vi "BoxExecute_ForSim.vi"(11 "Inputs":T5) -> (1 "OtherOutputs":T3={"ShootLOnTarg"=FALSE, "ShootROnTarg"=FALSE, "StateMachineState"=enum."initilization", "Box Note State"=enum."note in shooter wheels", "ShootR SP"=0.0, "ShootR FF"=0.0, "ShootR Filt RPM"=0.0, "ShootL SP"=0.0, "ShootL FF"=0.0, "ShootL Filt RPM"=0.0}, 3 "Outputs":T4)   [LabVIEW 2023]
uses:
  BoxStatesEnum.ctl
  BoxNoteState.ctl
  <vilib>/Rock Robotics/WPI/ThirdParty/JAS_Junk/TrajLib/TypeDef/PID_ERROR_TOLERANCE.ctl
  <vilib>/Rock Robotics/WPI/ThirdParty/JAS_Junk/TrajLib/LinearFilter_ResetToValue.vi
  <vilib>/Rock Robotics/WPI/ThirdParty/JAS_Junk/TrajLib/LinearFilter_Calculate.vi
  <vilib>/Rock Robotics/WPI/ThirdParty/JAS_Junk/TrajLib/VI/BoolCmd_Recv_Internal.vi
  <vilib>/Rock Robotics/WPI/ThirdParty/JAS_Junk/TrajLib/VI/DigSeqLogic_Edge_On.vi
  <vilib>/Rock Robotics/WPI/ThirdParty/JAS_Junk/TrajLib/SimpleMotorFF_Calculate.vi
  <vilib>/Rock Robotics/WPI/ThirdParty/JAS_Junk/TrajLib/PIDController_AtSetpoint.vi
  <vilib>/Rock Robotics/WPI/ThirdParty/JAS_Junk/TrajLib/PIDController_SetPIDF.vi
  <vilib>/Rock Robotics/WPI/ThirdParty/JAS_Junk/TrajLib/PIDController_SetDerivativeFilter.vi
  <vilib>/Rock Robotics/WPI/ThirdParty/JAS_Junk/TrajLib/PIDController_SetIntegratorRange.vi
  <vilib>/Rock Robotics/WPI/ThirdParty/JAS_Junk/TrajLib/PIDController_SetTolerancePandV.vi
  <vilib>/Rock Robotics/WPI/ThirdParty/JAS_Junk/TrajLib/PIDController_DisableContinousInput.vi
  <vilib>/Rock Robotics/WPI/ThirdParty/JAS_Junk/TrajLib/PIDController_EnableContinousInput.vi
  <vilib>/Rock Robotics/WPI/ThirdParty/JAS_Junk/TrajLib/PIDController_Reset.vi
  <vilib>/Rock Robotics/WPI/ThirdParty/JAS_Junk/TrajLib/PIDController_New.vi
  <vilib>/Rock Robotics/WPI/ThirdParty/JAS_Junk/TrajLib/PIDController_SetOutputLimits.vi
  <vilib>/Rock Robotics/WPI/ThirdParty/JAS_Junk/TrajLib/VI/BoolCmd_ObtainQueue.vi
  <vilib>/Rock Robotics/WPI/ThirdParty/JAS_Junk/TrajLib/PIDController_NewPeriod.vi
  <vilib>/Rock Robotics/SystemInterfaces/NetworkCommunication/NetComm_UsageReport_report.vi
  BoxGlobals.vi
  <vilib>/Rock Robotics/Network Tables/NT Write Boolean.vi
  <vilib>/Rock Robotics/WPI/ThirdParty/JAS_Junk/TrajLib/LinearFilter_MovingAverage.vi
  <vilib>/Rock Robotics/WPI/ThirdParty/JAS_Junk/TrajLib/LinearFilter_LowPassBW1.vi
  <vilib>/Rock Robotics/WPI/ThirdParty/JAS_Junk/TrajLib/LinearFilter_LowPassBW2.vi
  <vilib>/Rock Robotics/WPI/ThirdParty/JAS_Junk/TrajLib/LinearFilter_HighPassBW1.vi
  <vilib>/Rock Robotics/WPI/ThirdParty/JAS_Junk/TrajLib/LinearFilter_HighPassBW2.vi
  <vilib>/Rock Robotics/Network Tables/NT Write Number.vi
  <vilib>/Rock Robotics/Network Tables/NT Write String.vi
  <vilib>/Utility/semaphor.llb/Obtain Semaphore Reference.vi
  <vilib>/Rock Robotics/WPI/ThirdParty/JAS_Junk/TrajLib/Timer_Reset.vi
  <vilib>/Rock Robotics/WPI/ThirdParty/JAS_Junk/TrajLib/Timer_Start.vi
  <vilib>/Rock Robotics/WPI/ThirdParty/JAS_Junk/TrajLib/Timer_Stop.vi
  <vilib>/Rock Robotics/WPI/ThirdParty/JAS_Junk/TrajLib/Globals/Util_LibraryGlobals.vi
  <vilib>/Rock Robotics/WPI/ThirdParty/JAS_Junk/TrajLib/PIDController_AdvCalculate_FF_Sp_Pv.vi
  <vilib>/Rock Robotics/WPI/ThirdParty/JAS_Junk/TrajLib/Trajectory_Library.lvlib
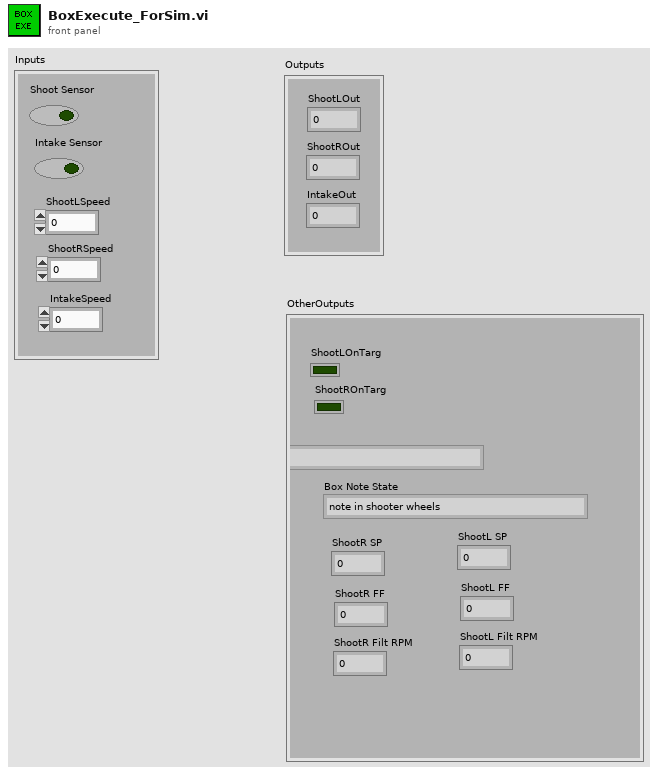
[diagram p1: front panel]
types:
  T1 = typedef "BoxStatesEnum.ctl" = enum16{"get input", "start shoot wheels", "up to speed?", "run intake", "have ring?", "stop intake and shooter", "start intake", "pick up ring or  _ sec?", "stop intake", "start source  intake", "pick up note?", "stop intake shooter", "shoot amp", "used note?", "stop amp intake", "initilization"}
  T2 = typedef "BoxNoteState.ctl" = enum16{"note in shooter wheels", "misaligned note", "no note", "have note"}
  T3 = cluster{"ShootLOnTarg":bool, "ShootROnTarg":bool, "StateMachineState":T1, "Box Note State":T2, "ShootR SP":dbl, "ShootR FF":dbl, "ShootR Filt RPM":dbl, "ShootL SP":dbl, "ShootL FF":dbl, "ShootL Filt RPM":dbl}
  T4 = cluster{"ShootLOut":dbl, "ShootROut":dbl, "IntakeOut":dbl}
  T5 = cluster{"Shoot Sensor":bool, "Intake Sensor":bool, "ShootLSpeed":dbl, "ShootRSpeed":dbl, "IntakeSpeed":dbl}
  T6 = enum16{"Moving Average", "Low Pass 1st Order Butterworth", "Low Pass 2nd Order Butterworth", "High Pass 1st Order Butterworth", "High Pass 2nd Order Butterworth"}
  T7 = typedef "Trajectory_Library.lvlib/PID_ERROR_TOLERANCE.ctl" = cluster{"PositionTolerance":dbl, "VelocityTolerance":dbl}
  T8 = typedef "Trajectory_Library.lvlib/SIMPLE_MOTOR_FF.ctl" = cluster{"Ks":dbl, "Kv":dbl, "Ka":dbl, "KnInv":dbl}
  T9 = typedef "Trajectory_Library.lvlib/TIMER.ctl" = cluster{"StartTime":dbl, "Accumulated TIme":dbl, "Running":bool, "semaphore":T10}
  T10 = typedef "Semaphore RefNum" = refnum<k1>
  T11 = typedef "Trajectory_Library.lvlib/PID_ADV_LIMITS.ctl" = cluster{"MaxInput":dbl, "MinInput":dbl, "Continuous":bool, "MaxOutput":dbl, "MinOutput":dbl}
  T12 = typedef "Trajectory_Library.lvlib/PID_ADV_TUNING.ctl" = cluster{"Kf":dbl, "Kp":dbl, "Ki":dbl, "Kd":dbl, "MaximumIntegral":dbl, "MinimumIntegral":dbl, "Filter Derivative":bool}
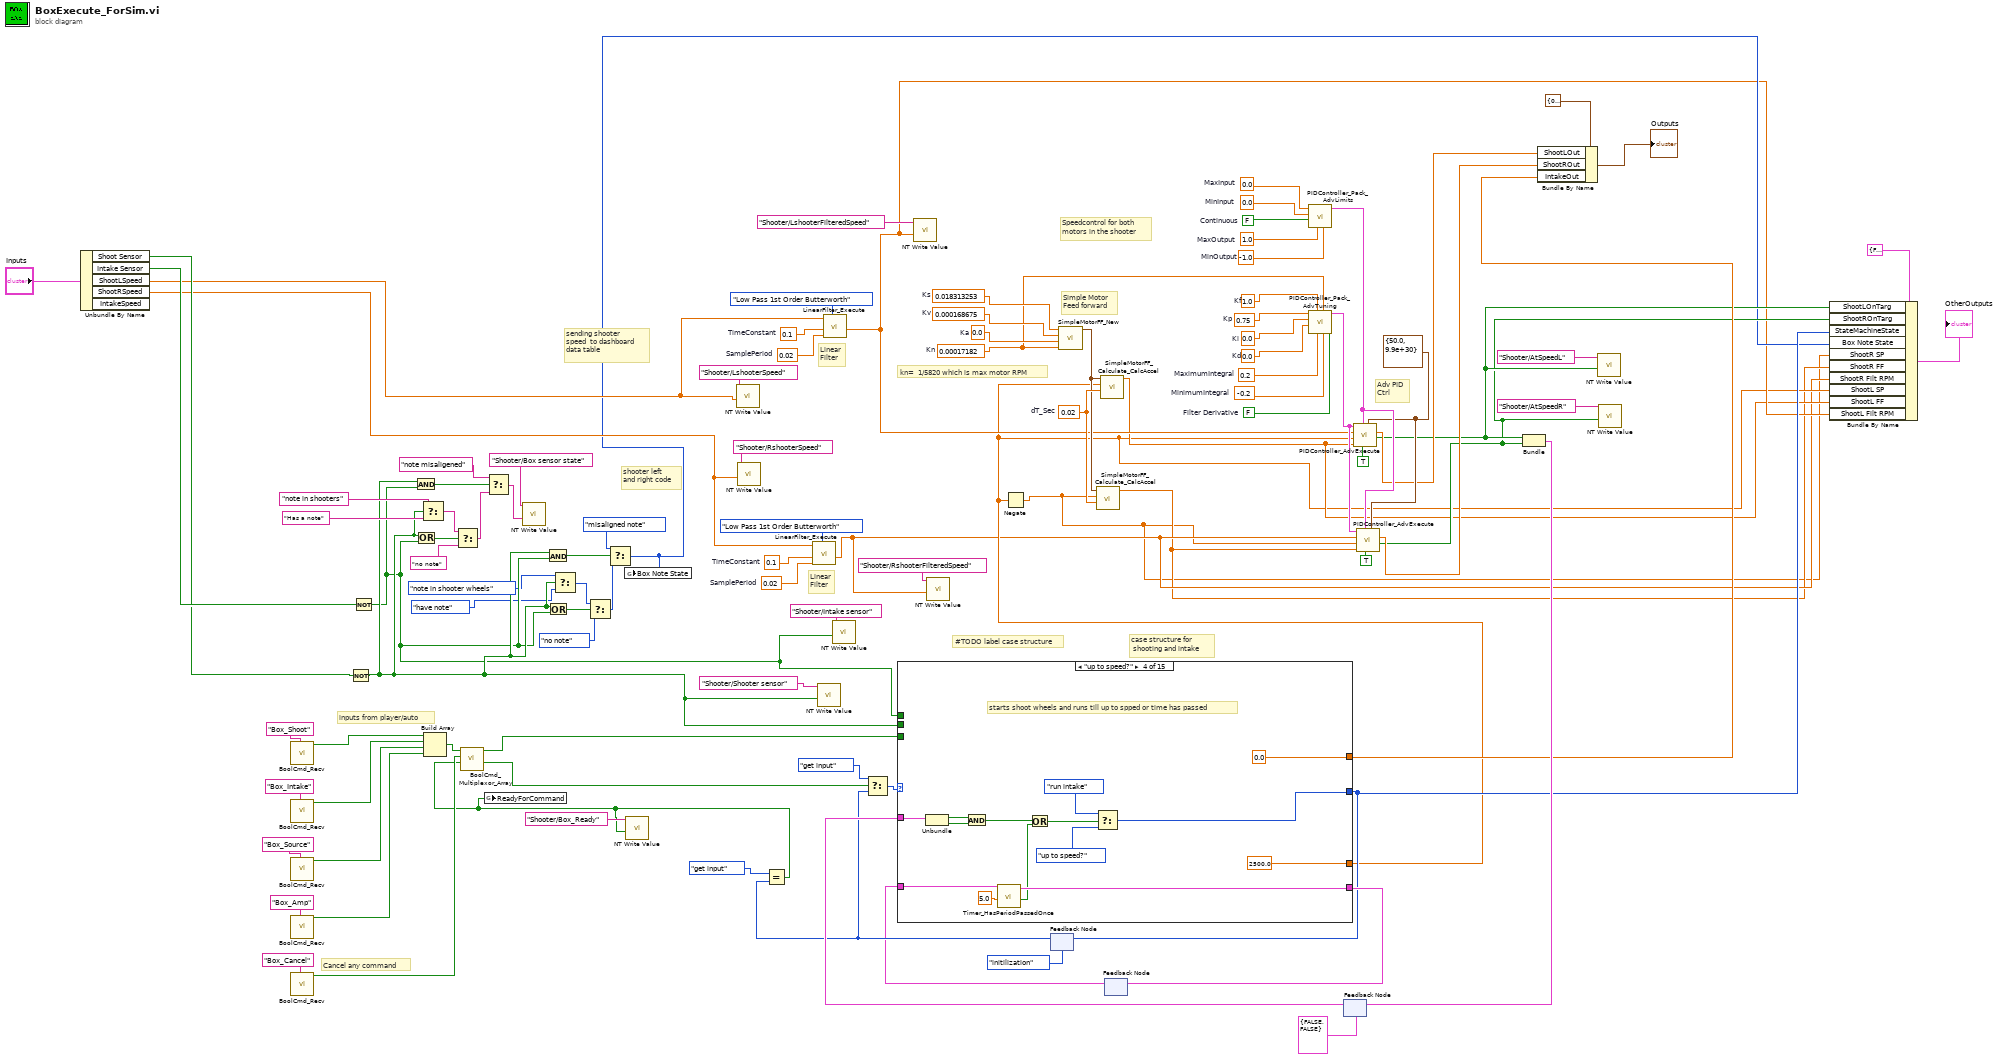
[diagram p0: block diagram]
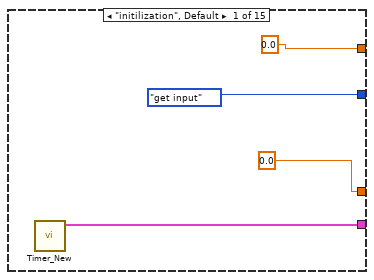
[diagram p2: hidden frame]
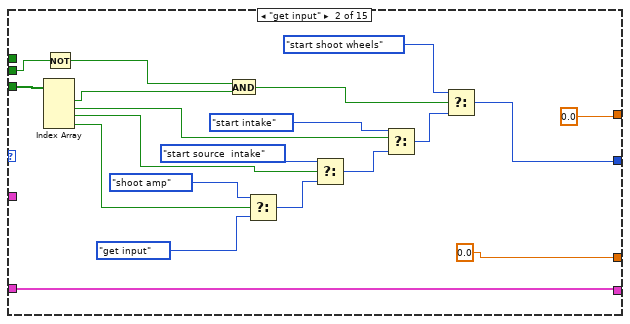
[diagram p3: hidden frame]
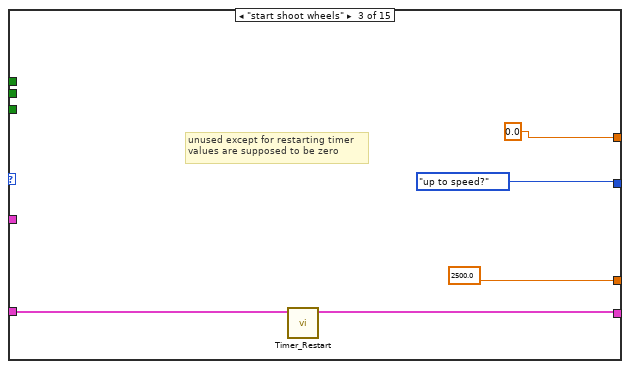
[diagram p4: hidden frame]
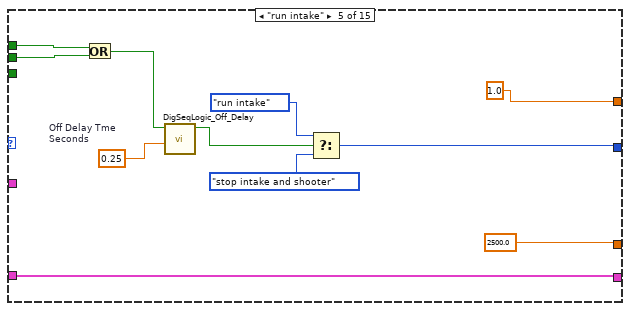
[diagram p5: hidden frame]
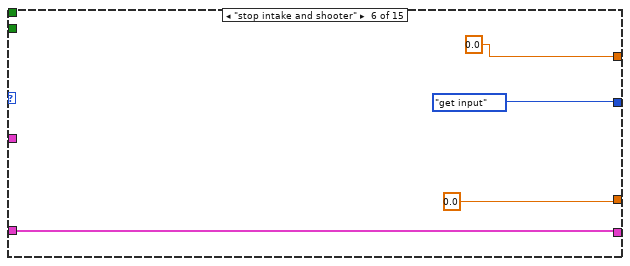
[diagram p6: hidden frame]
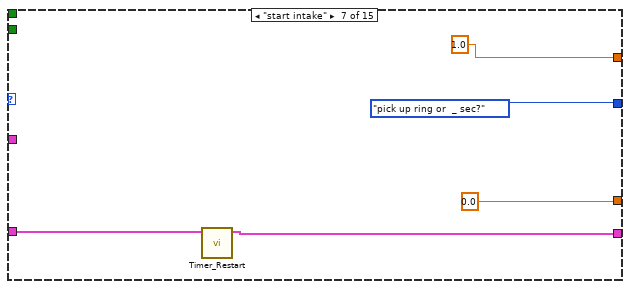
[diagram p7: hidden frame]
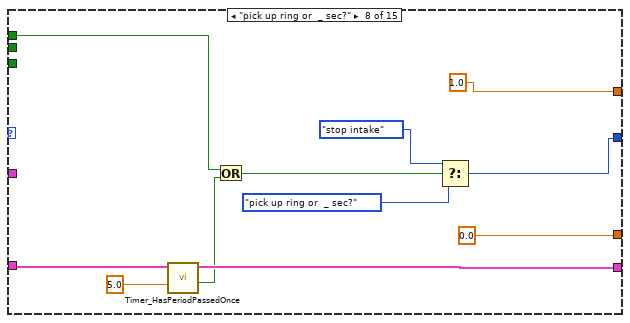
[diagram p8: hidden frame]
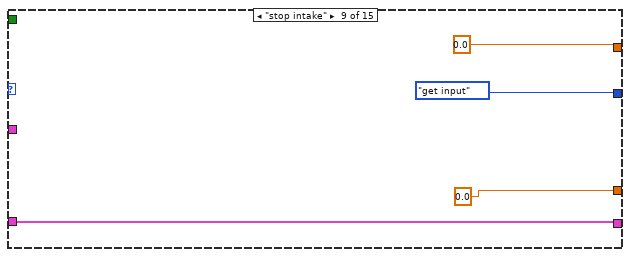
[diagram p9: hidden frame]
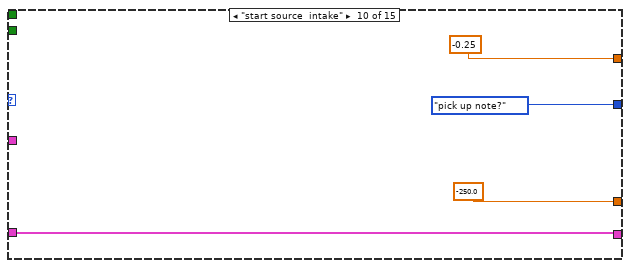
[diagram p10: hidden frame]
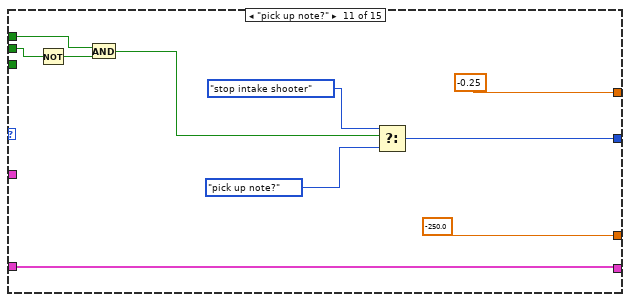
[diagram p11: hidden frame]
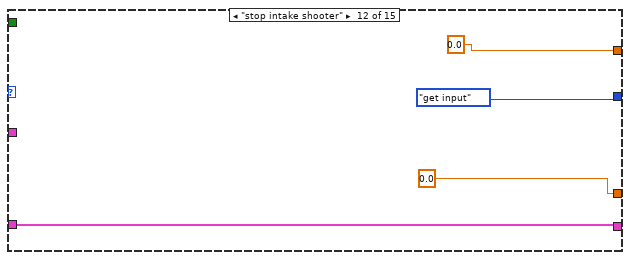
[diagram p12: hidden frame]
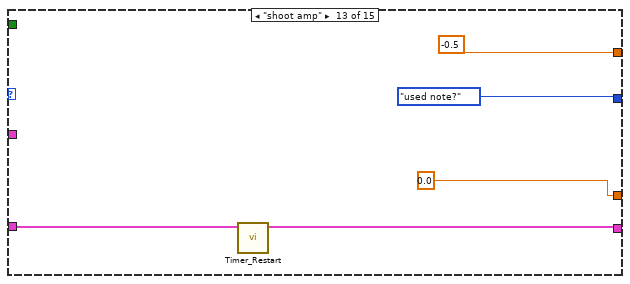
[diagram p13: hidden frame]
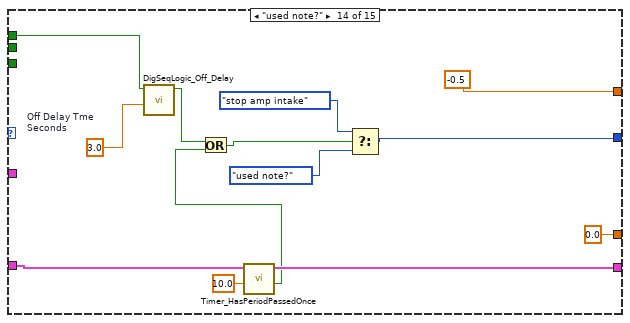
[diagram p14: hidden frame]
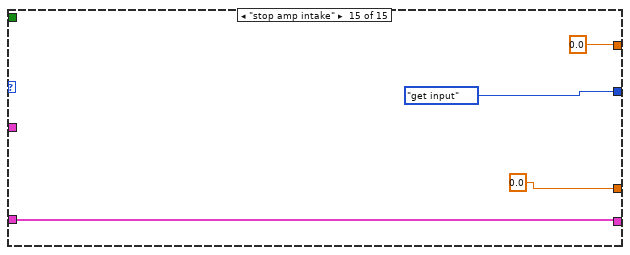
[diagram p15: hidden frame]
diagram:
  w54 = 0.02  # SamplePeriod
  w53 = 0.1  # TimeConstant
  w57 = 0.02  # SamplePeriod
  w56 = 0.1  # TimeConstant
  w60 = T7 {"PositionTolerance"=50.0, "VelocityTolerance"=9.9e+30} ("PID Error Tolerance")
  w73 = 0.00017182  # Kn
  w76 = 0.018313253  # Ks
  w75 = 0.000168675  # Kv
  w74 = 0.0  # Ka
  w71 = 0.75  # Kp
  w70 = 0.0  # Ki
  w69 = 0.0  # Kd
  w72 = 1.0  # Kf
  w68 = 0.2  # MaximumIntegral
  w67 = -0.2  # MinimumIntegral
  w66 = FALSE  # Filter Derivative
  w80 = 0.0  # MinInput
  w79 = FALSE  # Continuous
  w78 = 1.0  # MaxOutput
  w77 = -1.0  # MinOutput
  w81 = 0.0  # MaxInput
  w64 = 0.02  # dT_Sec
  # "#TODO label case structure"
  # "inputs from player/auto"
  # "Linear\nFilter"
  # "Linear\nFilter"
  # "Speedcontrol for both \nmotors in the shooter"
  # "Simple Motor\nFeed forward"
  # "Adv PID\nCtrl"
  # "Cancel any command"
  # "kn=  1/5820 which is max motor RPM"
  # "case structure for\n shooting and intake"
  # "sending shooter \nspeed  to dashboard \ndata table"
  # "shooter left \nand right code"
  n1 = Unbundle By Name("Inputs") -> ("Shoot Sensor"=w20:bool, "Intake Sensor"=w21:bool, "ShootLSpeed"=w19:dbl, "ShootRSpeed"=w18:dbl)  [unwired: 1 out]
  n2 = call <vilib>:"BoolCmd_Recv.vi"("Command Name"="Box_Shoot") -> ("New Request"=w95:bool)  [unwired: 9 in, 1 out]
  n3 = call <vilib>:"BoolCmd_Recv.vi"("Command Name"="Box_Intake") -> ("New Request"=w96:bool)  [unwired: 9 in, 1 out]
  n4 = call <vilib>:"BoolCmd_Recv.vi"("Command Name"="Box_Source") -> ("New Request"=w99:bool)  [unwired: 9 in, 1 out]
  n5 = call <vilib>:"BoolCmd_Recv.vi"("Command Name"="Box_Amp") -> ("New Request"=w100:bool)  [unwired: 9 in, 1 out]
  n6 = call <vilib>:"BoolCmd_Recv.vi"("Command Name"="Box_Cancel") -> ("New Request"=w93:bool)  [unwired: 9 in, 1 out]
  n7 = Not(x=w20) -> (.not. x?=w30:bool)
  n8 = Not(x=w21) -> (.not. x?=w29:bool)
  n9 = And(x=w30, y=w29) -> (x .and. y?=w45:bool)
  n10 = Or(x=w30, y=w29) -> (x .or. y?=w44:bool)
  n11 = Select(t="note in shooters", s=w30, f="Has a note") -> (s? t:f=w43:string)
  n12 = Build Array(w95, w96, w99, w100) -> (w94:bool[])
  n13 = Select(t=w43, s=w44, f="no note") -> (s? t:f=w41:string)
  n14 = Select(t="note misaligened", s=w45, f=w41) -> (s? t:f=w37:string)
  n15 = call-poly <vilib>:"NT Write Value.vi"("value"=w37, "name"="Shooter/Box sensor state") -> ()  [unwired: 9 in, 1 out]
  n16 = And(x=w30, y=w29) -> (x .and. y?=w34:bool)
  n17 = Or(x=w30, y=w29) -> (x .or. y?=w33:bool)
  n18 = Select(t=BoxNoteState."note in shooter wheels" ("Box Note State"), s=w30, f=BoxNoteState."have note" ("Box Note State")) -> (s? t:f=w32:T2)
  n19 = Select(t=w32, s=w33, f=BoxNoteState."no note" ("Box Note State")) -> (s? t:f=w31:T2)
  n20 = Select(t=BoxNoteState."misaligned note" ("Box Note State"), s=w34, f=w31) -> (s? t:f=w9:T2)
  n21 = global write "BoxGlobals.vi" "Box Note State"(w9) -> ()
  n22 = call-poly <vilib>:"NT Write Value.vi"("value"=w19, "name"="Shooter/LshooterSpeed") -> ()  [unwired: 9 in, 1 out]
  n23 = call-poly <vilib>:"NT Write Value.vi"("value"=w18, "name"="Shooter/RshooterSpeed") -> ()  [unwired: 9 in, 1 out]
  n24 = call <vilib>:"LinearFilter_Execute.vi"("Filter Type"=T6."Low Pass 1st Order Butterworth", "SamplePeriod"=w57, "TimeConstant"=w56, "Input"=w18) -> ("Output"=w3:dbl)  [unwired: 6 in, 1 out]
  n25 = call-poly <vilib>:"NT Write Value.vi"("value"=w30, "name"="Shooter/Shooter sensor") -> ()  [unwired: 9 in, 1 out]
  n26 = call <vilib>:"LinearFilter_Execute.vi"("Filter Type"=T6."Low Pass 1st Order Butterworth", "SamplePeriod"=w54, "TimeConstant"=w53, "Input"=w19) -> ("Output"=w6:dbl)  [unwired: 6 in, 1 out]
  n27 = call-poly <vilib>:"NT Write Value.vi"("value"=w29, "name"="Shooter/Intake sensor") -> ()  [unwired: 9 in, 1 out]
  n28 = call-poly <vilib>:"NT Write Value.vi"("value"=w6, "name"="Shooter/LshooterFilteredSpeed") -> ()  [unwired: 9 in, 1 out]
  n29 = call-poly <vilib>:"NT Write Value.vi"("value"=w3, "name"="Shooter/RshooterFilteredSpeed") -> ()  [unwired: 9 in, 1 out]
  n30 = feedback #1(BoxStatesEnum."initilization") -> (w85:T1)
  n31 = Equal?(x=BoxStatesEnum."get input" ("Box states"), y=w85) -> (x = y?=w35:bool)
  n32 = call <vilib>:"BoolCmd_Multiplexor_Array.vi"("Ready"=w35, "Command Cancel"=w93, "Commands"=w94) -> ("Do Cancel"=w87:bool, "Do Command"=w89:bool[])  [unwired: 7 in]
  n33 = global write "BoxGlobals.vi" "ReadyForCommand"(w35) -> ()
  n34 = call-poly <vilib>:"NT Write Value.vi"("value"=w35, "name"="Shooter/Box_Ready") -> ()  [unwired: 9 in, 1 out]
  n35 = Select(t=BoxStatesEnum."get input" ("Box states"), s=w87, f=w85) -> (s? t:f=w88:T1)
  n36 = call <vilib>:"SimpleMotorFF_New.vi"("Kn"=w73, "Ka"=w74, "Kv"=w75, "Ks"=w76) -> ("SIMPLE_MOTOR_FF"=w63:T8)  [unwired: 7 in]
  n37 = feedback #2() -> (w48:T9)  [unwired: 1 in]
  n38 = call <vilib>:"PIDController_Pack_AdvLimits.vi"("MinOutput"=w77, "MaxOutput"=w78, "Continuous"=w79, "MinInput"=w80, "MaxInput"=w81) -> ("Adv PID Limits"=w61:T11)  [unwired: 6 in]
  n39 = call <vilib>:"PIDController_Pack_AdvTuning.vi"("Filter Derivative"=w66, "MinimumIntegral"=w67, "Kn"=w73, "MaximumIntegral"=w68, "Kf"=w72, "Kd"=w69, "Ki"=w70, "Kp"=w71) -> ("Adv PID Tuning"=w62:T12)  [unwired: 3 in]
  n40 = feedback #3(cluster{bool, bool} {FALSE, FALSE}) -> (w101:cluster{bool, bool})
  n41 = case shown="\"up to speed?\"" w88 {
    tunnel: [BoxStatesEnum."get input" ("Box states") w121 BoxStatesEnum."up to speed?" ("Box states") w142 w154 BoxStatesEnum."get input" ("Box states") BoxStatesEnum."pick up ring or  _ sec?" ("Box states") w174 BoxStatesEnum."get input" ("Box states") BoxStatesEnum."pick up note?" ("Box states") w191 BoxStatesEnum."get input" ("Box states") BoxStatesEnum."used note?" ("Box states") w214 BoxStatesEnum."get input" ("Box states")] -> w10
    tunnel: w101 -> [_ _ _ w145 _ _ _ _ _ _ _ _ _ _ _]
    tunnel: [0.0 0.0 2500.0 2500.0 2500.0 0.0 0.0 0.0 0.0 -250.0 -250.0 0.0 0.0 0.0 0.0] -> w4
    tunnel: [0.0 0.0 0.0 0.0 1.0 0.0 1.0 1.0 0.0 -0.25 -0.25 0.0 -0.5 -0.5 0.0] -> w13
    tunnel: w89 -> [_ w127 _ _ _ _ _ _ _ _ _ _ _ _ _]
    tunnel: w29 -> [_ _ _ _ w153 _ _ w173 _ _ w189 _ _ w207 _]
    tunnel: w30 -> [_ w110 _ _ w152 _ _ _ _ _ w190 _ _ _ _]
    tunnel: [w105 w113 w129 w138 w151 w159 w164 w169 w179 w183 w194 w197 w201 w212 w219] -> w49
    tunnel: w48 -> [_ w113 w130 w139 w151 w159 w163 w171 w179 w183 w194 w197 w202 w213 w219]
    frame "initilization", Default {
      n42 = call <vilib>:"Timer_New.vi"() -> ("TIMER"=w105:T9)  [unwired: 11 in]
    }
    frame "get input" {
      n43 = Index Array(array=w127) -> (element #1=w111:bool, element #2=w118:bool, element #3=w117:bool, element #4=w116:bool)  [unwired: 4 in]
      n44 = Not(x=w110) -> (.not. x?=w109:bool)
      n45 = And(x=w109, y=w111) -> (x .and. y?=w112:bool)
      n46 = Select(t=BoxStatesEnum."shoot amp" ("Box states"), s=w116, f=BoxStatesEnum."get input" ("Box states")) -> (s? t:f=w122:T1)
      n47 = Select(t=BoxStatesEnum."start source  intake", s=w117, f=w122) -> (s? t:f=w123:T1)
      n48 = Select(t=BoxStatesEnum."start intake" ("Box states"), s=w118, f=w123) -> (s? t:f=w124:T1)
      n49 = Select(t=BoxStatesEnum."start shoot wheels" ("Box states"), s=w112, f=w124) -> (s? t:f=w121:T1)
    }
    frame "start shoot wheels" {
      # "unused except for restarting timer\nvalues are supposed to be zero"
      n50 = call <vilib>:"Timer_Restart.vi"("in Timer"=w130) -> ("out Timer"=w129:T9)  [unwired: 10 in]
    }
    frame "up to speed?" {
      # "starts shoot wheels and runs till up to spped or time has passed"
      n51 = Unbundle(w145) -> (w144:bool, w143:bool)
      n52 = And(x=w144, y=w143) -> (x .and. y?=w136:bool)
      n53 = call <vilib>:"Timer_HasPeriodPassedOnce.vi"("Period"=5.0, "in Timer"=w139) -> ("Expired"=w134:bool, "out Timer"=w138:T9)  [unwired: 7 in, 1 out]
      n54 = Or(x=w136, y=w134) -> (x .or. y?=w135:bool)
      n55 = Select(t=BoxStatesEnum."run intake" ("Box states"), s=w135, f=BoxStatesEnum."up to speed?" ("Box states")) -> (s? t:f=w142:T1)
    }
    frame "run intake" {
      w150 = 0.25  # Off Delay Tme Seconds
      n56 = Or(x=w153, y=w152) -> (x .or. y?=w149:bool)
      n57 = call <vilib>:"DigSeqLogic_Off_Delay.vi"("Delay"=w150, "Input"=w149) -> ("Output"=w148:bool)  [unwired: 8 in, 1 out]
      n58 = Select(t=BoxStatesEnum."run intake" ("Box states"), s=w148, f=BoxStatesEnum."stop intake and shooter" ("Box states")) -> (s? t:f=w154:T1)
    }
    frame "stop intake and shooter" {
    }
    frame "start intake" {
      n59 = call <vilib>:"Timer_Restart.vi"("in Timer"=w163) -> ("out Timer"=w164:T9)  [unwired: 10 in]
    }
    frame "pick up ring or  _ sec?" {
      n60 = call <vilib>:"Timer_HasPeriodPassedOnce.vi"("Period"=5.0, "in Timer"=w171) -> ("Expired"=w168:bool, "out Timer"=w169:T9)  [unwired: 7 in, 1 out]
      n61 = Or(x=w173, y=w168) -> (x .or. y?=w172:bool)
      n62 = Select(t=BoxStatesEnum."stop intake" ("Box states"), s=w172, f=BoxStatesEnum."pick up ring or  _ sec?" ("Box states")) -> (s? t:f=w174:T1)
    }
    frame "stop intake" {
    }
    frame "start source  intake" {
    }
    frame "pick up note?" {
      n63 = Not(x=w190) -> (.not. x?=w188:bool)
      n64 = And(x=w189, y=w188) -> (x .and. y?=w187:bool)
      n65 = Select(t=BoxStatesEnum."stop intake shooter" ("Box states"), s=w187, f=BoxStatesEnum."pick up note?" ("Box states")) -> (s? t:f=w191:T1)
    }
    frame "stop intake shooter" {
    }
    frame "shoot amp" {
      n66 = call <vilib>:"Timer_Restart.vi"("in Timer"=w202) -> ("out Timer"=w201:T9)  [unwired: 10 in]
    }
    frame "used note?" {
      w208 = 3.0  # Off Delay Tme Seconds
      n67 = call <vilib>:"DigSeqLogic_Off_Delay.vi"("Delay"=w208, "Input"=w207) -> ("Output"=w206:bool)  [unwired: 8 in, 1 out]
      n68 = call <vilib>:"Timer_HasPeriodPassedOnce.vi"("Period"=10.0, "in Timer"=w213) -> ("Expired"=w210:bool, "out Timer"=w212:T9)  [unwired: 7 in, 1 out]
      n69 = Or(x=w206, y=w210) -> (x .or. y?=w209:bool)
      n70 = Select(t=BoxStatesEnum."stop amp intake" ("Box states"), s=w209, f=BoxStatesEnum."used note?" ("Box states")) -> (s? t:f=w214:T1)
    }
    frame "stop amp intake" {
    }
  }
  n71 = Negate(x=w4) -> (-x=w1:dbl)
  n72 = feedback-in #1(w10) -> ()
  n73 = call <vilib>:"SimpleMotorFF_Calculate_CalcAccel.vi"("dT_Sec"=w64, "VelSp"=w1, "SIMPLE_MOTOR_FF"=w63) -> ("FeedForward"=w2:dbl)  [unwired: 8 in]
  n74 = call <vilib>:"SimpleMotorFF_Calculate_CalcAccel.vi"("dT_Sec"=w64, "VelSp"=w4, "SIMPLE_MOTOR_FF"=w63) -> ("FeedForward"=w5:dbl)  [unwired: 8 in]
  n75 = feedback-in #2(w49) -> ()
  n76 = call <vilib>:"PIDController_AdvExecute.vi"("PID Error Tolerance"=w60, "Auto"=TRUE, "Adv PID Limits"=w61, "FF-FeedForward"=w5, "SP-SetPoint"=w4, "PV-Measurement"=w6, "Adv PID Tuning"=w62) -> ("AtSetpoint"=w12:bool, "CO-ControlOutput"=w15:dbl)  [unwired: 2 in, 1 out]
  n77 = call <vilib>:"PIDController_AdvExecute.vi"("PID Error Tolerance"=w60, "Auto"=TRUE, "Adv PID Limits"=w61, "FF-FeedForward"=w2, "SP-SetPoint"=w1, "PV-Measurement"=w3, "Adv PID Tuning"=w62) -> ("AtSetpoint"=w11:bool, "CO-ControlOutput"=w14:dbl)  [unwired: 2 in, 1 out]
  n78 = Bundle("AtSetpoint"=w12, "AtSetpoint"=w11) -> (w58:cluster{"AtSetpoint":bool, "AtSetpoint":bool})  [unwired: 1 in]
  n79 = feedback-in #3(w58) -> ()
  n80 = Bundle By Name(cluster=T4 {"ShootLOut"=0.0, "ShootROut"=0.0, "IntakeOut"=0.0} ("Outputs"), "ShootLOut"=w15, "ShootROut"=w14, "IntakeOut"=w13) -> (→"Outputs":T4)
  n81 = call-poly <vilib>:"NT Write Value.vi"("value"=w12, "name"="Shooter/AtSpeedL") -> ()  [unwired: 9 in, 1 out]
  n82 = call-poly <vilib>:"NT Write Value.vi"("value"=w11, "name"="Shooter/AtSpeedR") -> ()  [unwired: 9 in, 1 out]
  n83 = Bundle By Name(cluster=T3 {"ShootLOnTarg"=FALSE, "ShootROnTarg"=FALSE, "StateMachineState"=enum."initilization", "Box Note State"=enum."note in shooter wheels", "ShootR SP"=0.0, "ShootR FF"=0.0, "ShootR Filt RPM"=0.0, "ShootL SP"=0.0, "ShootL FF"=0.0, "ShootL Filt RPM"=0.0} ("OtherOutputs"), "ShootLOnTarg"=w12, "ShootROnTarg"=w11, "StateMachineState"=w10, "Box Note State"=w9, "ShootR SP"=w1, "ShootR FF"=w2, "ShootR Filt RPM"=w3, "ShootL SP"=w4, "ShootL FF"=w5, "ShootL Filt RPM"=w6) -> (→"OtherOutputs":T3)
